vi "ESP32 Continuous Serial Write and Read.vi"() -> ()   [LabVIEW 2021]
doc: "This example performs writes and reads on a serial port, as directed by the user. You can press the Write and Read buttons, and change the Read Count, while the example is running.\n\nThe parameters set for the serial port must match the parameters of the connected instrument or device. In this example, the Read Count parameter specifies the number of bytes that the serial port reads. If there were more bytes at the port than the specified number, those bytes would not be read. If there were less bytes at the port than the specified number, you would receive a timeout error.\n\nThis example expands upon the flow control options for XON and XOFF, allowing the user to choose those control characters. Also, the user can enable or disable a termination character. Some devices require a termination character in order to identify the end of command strings. Some devices send a termination character to signify the end of data to be read. This example shows how you can end the Read operation once a termination character is detected in the buffer and/or append a termination character at the end of the Write data."
uses:
  Program Files (x86)/National Instruments/LabVIEW 2021/examples/Instrument IO/Serial/support/Serial - Settings.ctl
  Program Files (x86)/National Instruments/LabVIEW 2021/examples/Instrument IO/Serial/support/Serial - XON-XOFF Characters.ctl
  Program Files (x86)/National Instruments/LabVIEW 2021/examples/Instrument IO/Serial/support/Serial - ASCII Characters.ctl
  ESP32-PSOC-State Machine.ctl
  <vilib>/Instr/_visa.llb/VISA Flush IO Buffer Mask.ctl
  <vilib>/Instr/_visa.llb/VISA Configure Serial Port (Instr).vi
panel:
  out "error":bool
  out "Connected":bool
  out "Serial Settings:Number of Bytes at Serial Port":u32
  out "Response 2":string
  in  "Command B":bool
  in  "Command A":bool
  in  "Toggle LED":bool
  in  "Enum":T1
  in  "Termination Character":u8=10 format="%.0x"
  in  "End Write on Termination Character?":bool=TRUE
  in  "Stop":bool
  out "Read Count":u32=1000
  out "Response":string
  in  "XON/XOFF Characters":T2={"XON"=enum."DC1", "XOFF"=enum."DC3"}
  in  "Serial Settings":T4={"baud rate"=115200, "data bits"=8, "parity"=enum."None", "stop bits"=10, "flow control"=0} {"flow control" items=["None"=0, "XON/XOFF"=1, "RTS/CTS"=2, "DTR/DSR"=4]; "stop bits" items=["1.0"=10, "1.5"=15, "2.0"=20]; "data bits" min=5 max=8 step=1; "baud rate" items=["75"=75, "110"=110, "134"=134, "150"=150, "300"=300, "600"=600, "1200"=1200, "1800"=1800, "2400"=2400, "4800"=4800, "7200"=7200, "9600"=9600, "14400"=14400, "19200"=19200, "28800"=28800, "38400"=38400, "56000"=56000, "57600"=57600, "115200"=115200, "128000"=128000, "230400"=230400]}
  in  "End Read on Termination Character?":bool=TRUE
  in  "VISA resource name":refnum<visa-resource-name>="COM4"
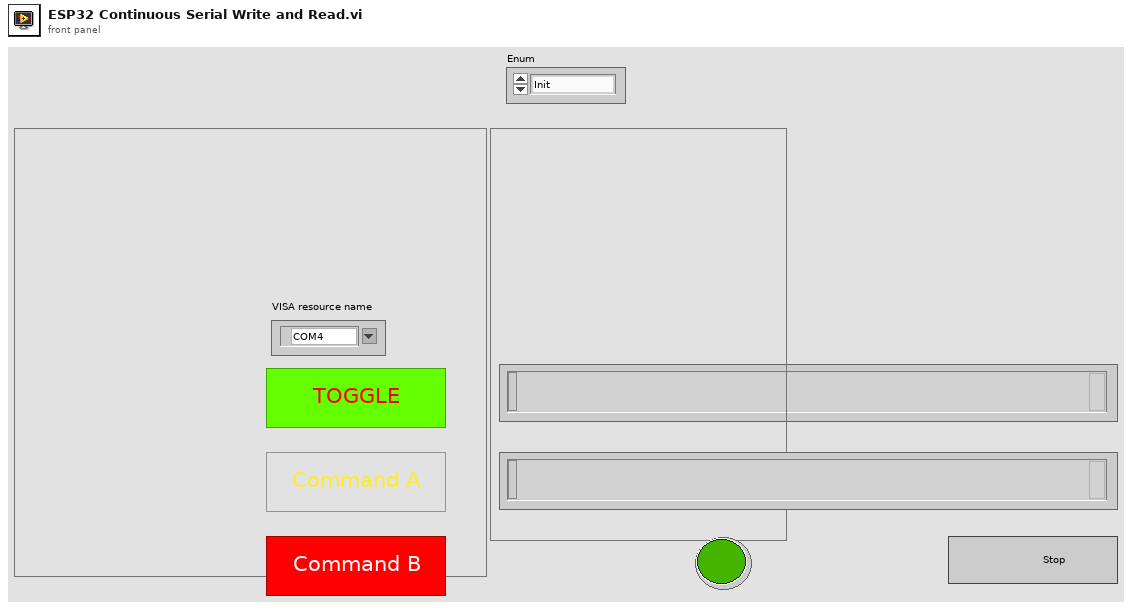
[diagram p1: front panel]
types:
  T1 = typedef "ESP32-PSOC-State Machine.ctl" = enum8{"Init", "Connect", "idle", "send", "wait", "receive", "que", "error", "exit"}
  T2 = typedef "Serial - XON-XOFF Characters.ctl" = cluster{"XON":T3, "XOFF":T3}
  T3 = typedef "Serial - ASCII Characters.ctl" = enum16{"NUL", "SOH", "STX", "ETX", "EOT", "ENQ", "ACK", "BEL", "BS", "HT", "LF", "VT", "FF", "CR", "SO", "SI", "DLE", "DC1", "DC2", "DC3", "DC4", "NAK", "SYN", "ETB", "CAN", "EM", "SUB", "ESC", "FS", "GS", "RS", "US", "SP", "!", "\"", "#", "$", "%", "&", "'", "(", ")", "*", "+", ",", "- (-)", ".", "/", "0", "1", "2", "3", "4", "5", "6", "7", "8", "9", ":", ";", "<", "=", ">", "?", "@", "A", "B", "C", "D", "E", "F", "G", "H", "I", "J", "K", "L", "M", "N", "O", "P", "Q", "R", "S", "T", "U", "V", "W", "X", "Y", "Z", "[", "\\", "]", "^", "_", "`", "a", "b", "c", "d", "e", "f", "g", "h", "i", "j", "k", "l", "m", "n", "o", "p", "q", "r", "s", "t", "u", "v", "w", "x", "y", "z", "{", "|", "}", "~"}
  T4 = typedef "Serial - Settings.ctl" = cluster{"baud rate":u32, "data bits":u16, "parity":enum16{"None", "Odd", "Even", "Mark", "Space"}, "stop bits":u16, "flow control":u16}
  T5 = typedef "VISA Flush IO Buffer Mask.ctl" = u16
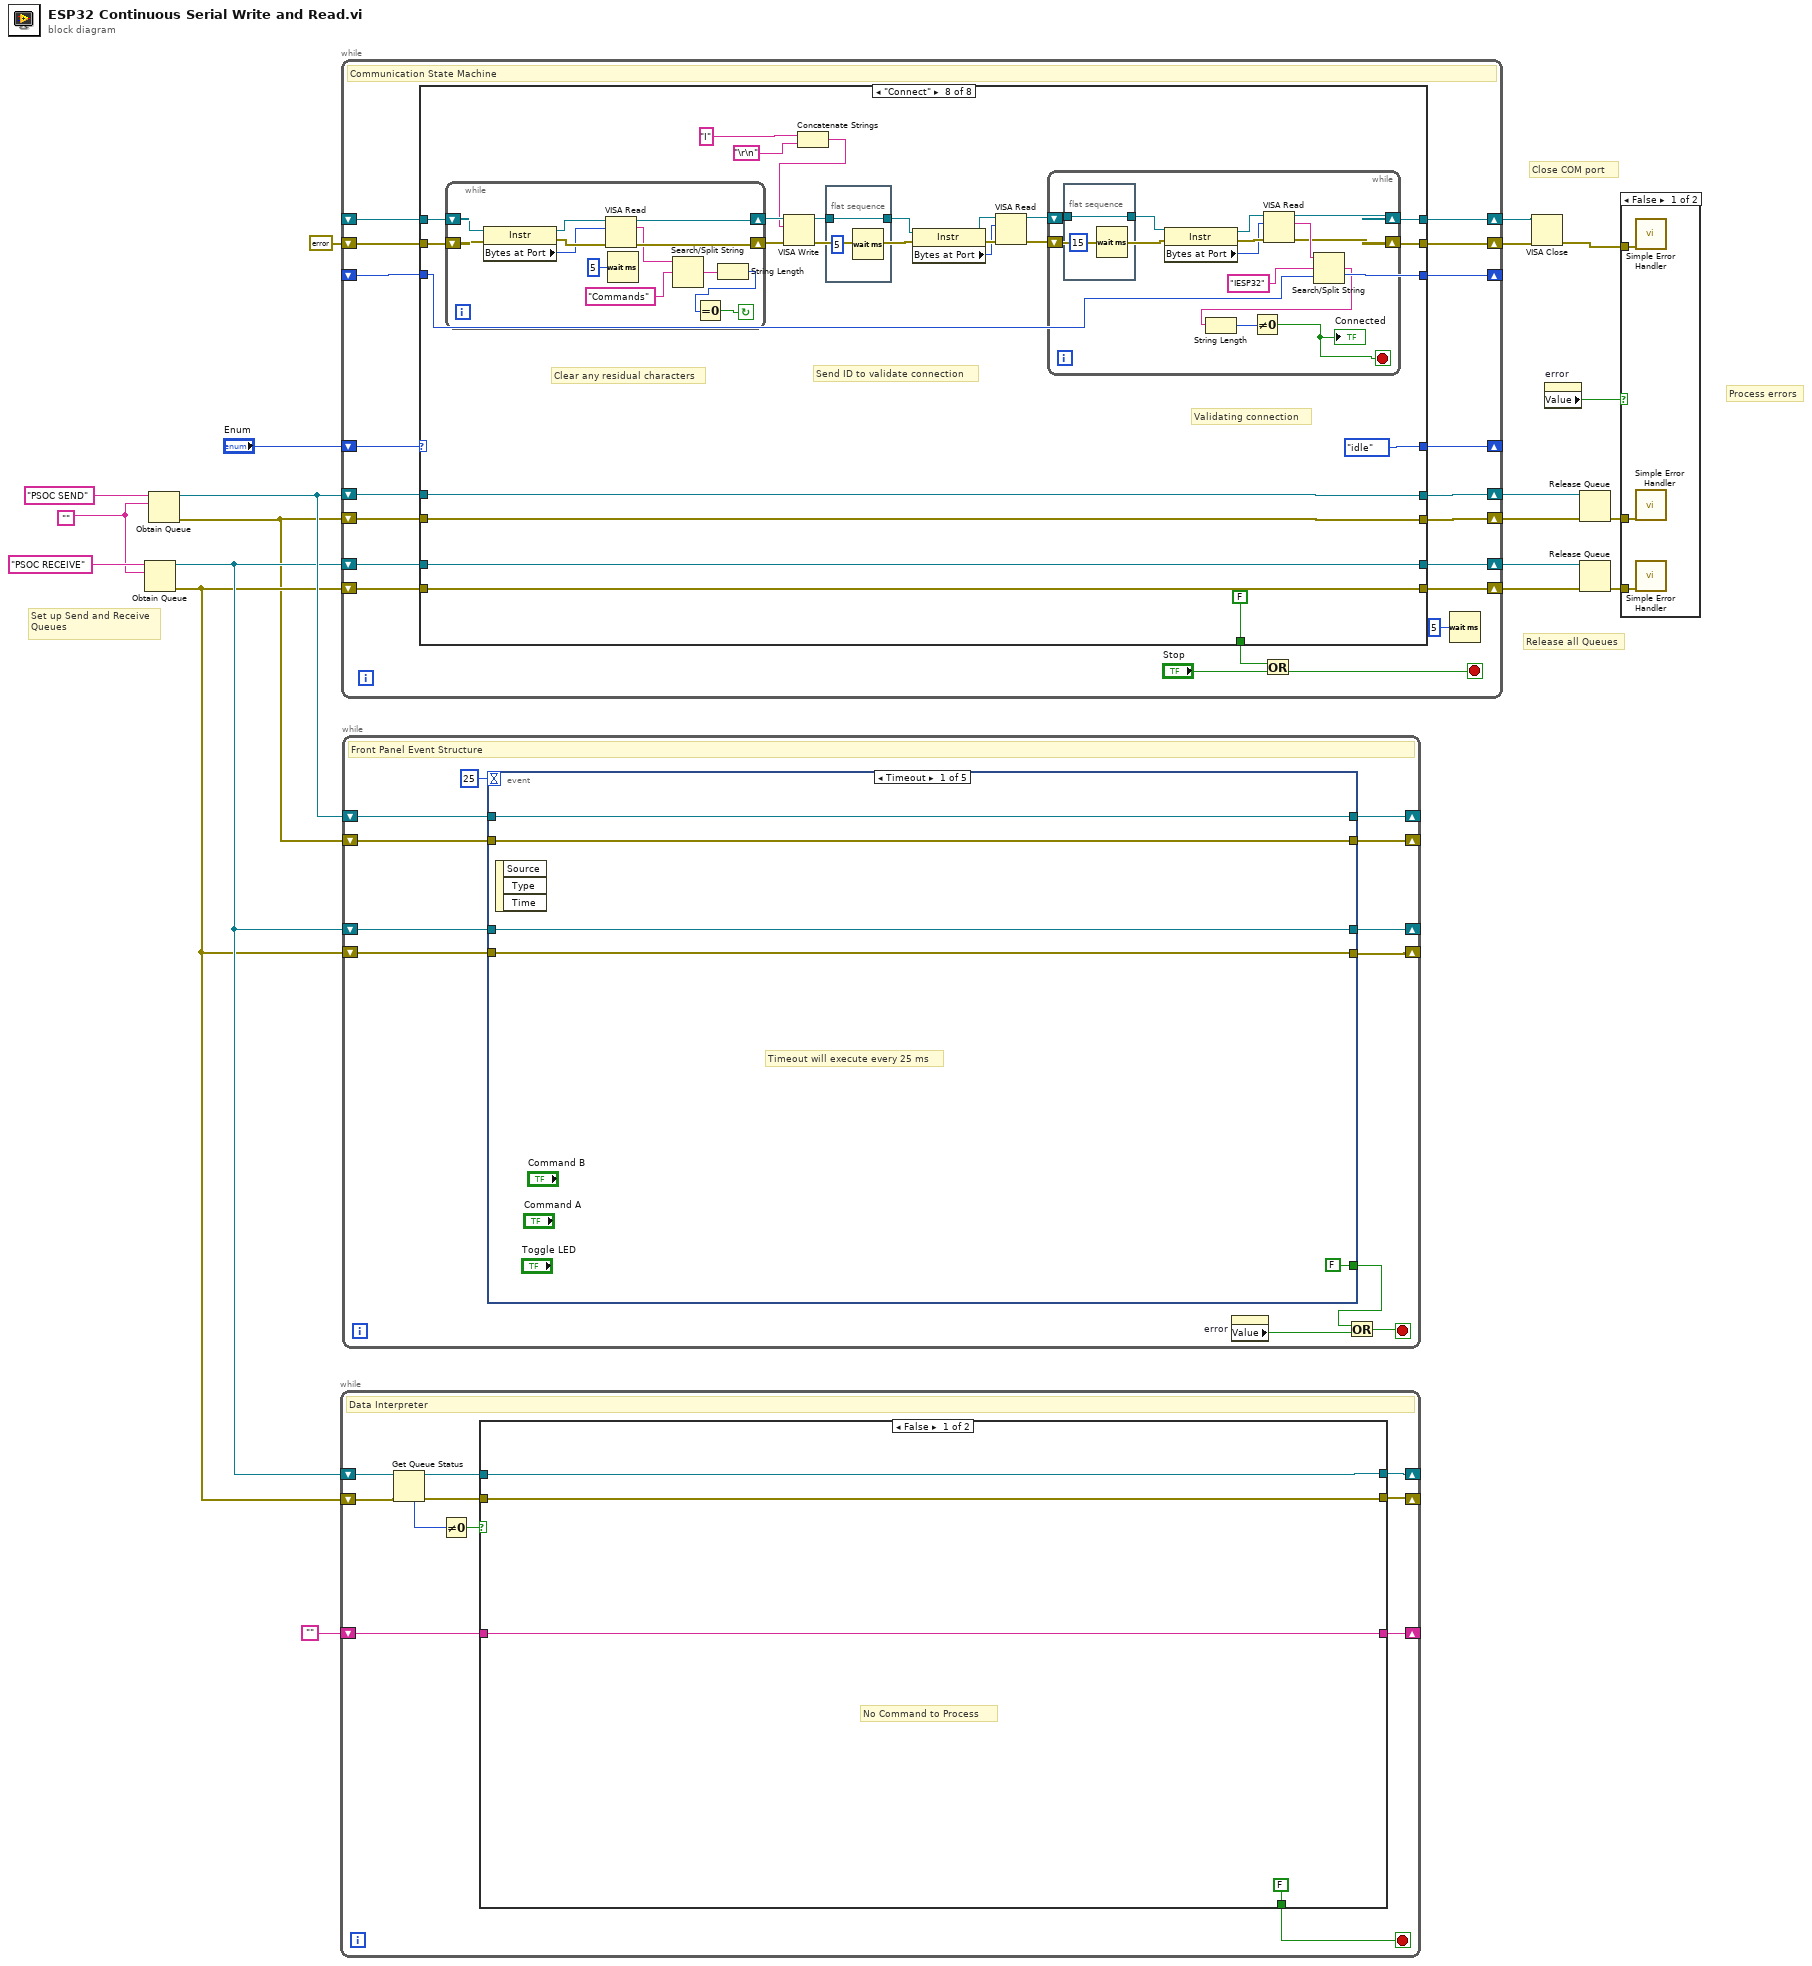
[diagram p0: block diagram]
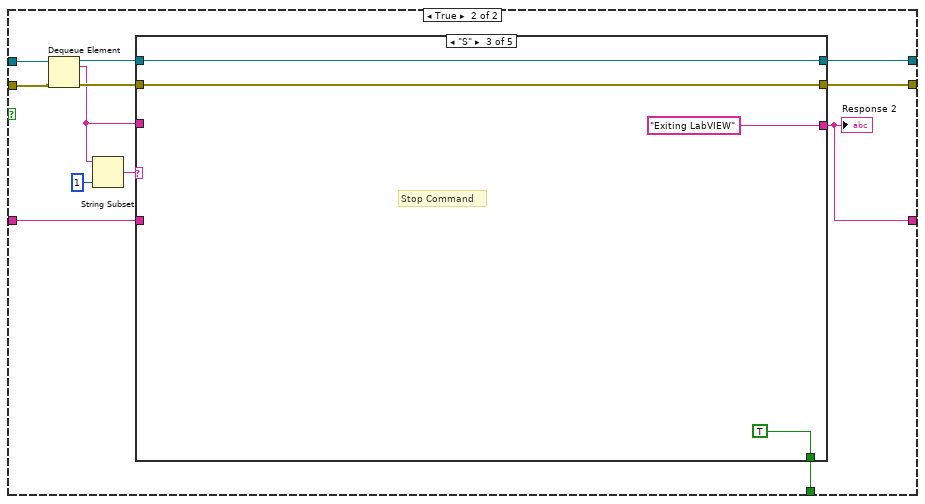
[diagram p3: hidden frame]
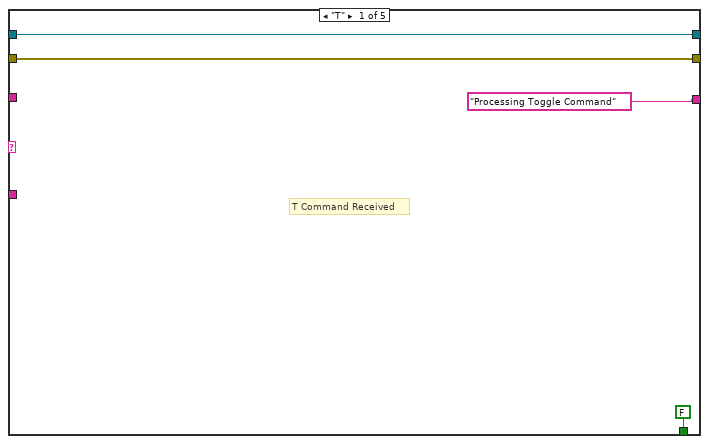
[diagram p4: hidden frame]
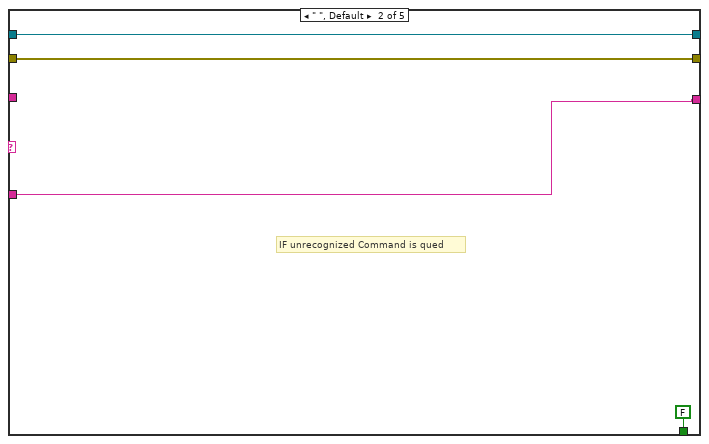
[diagram p5: hidden frame]
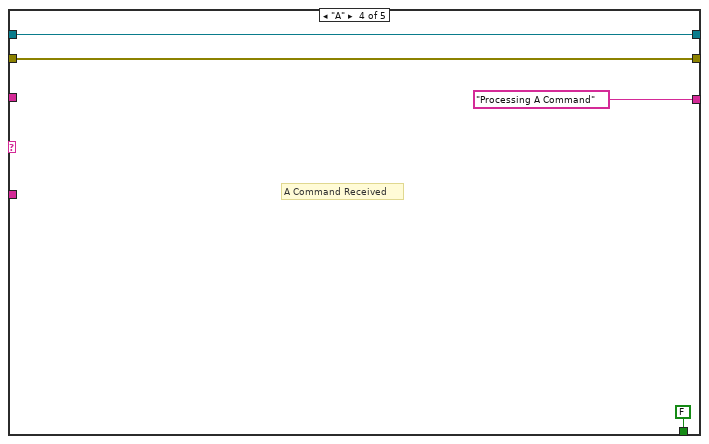
[diagram p6: hidden frame]
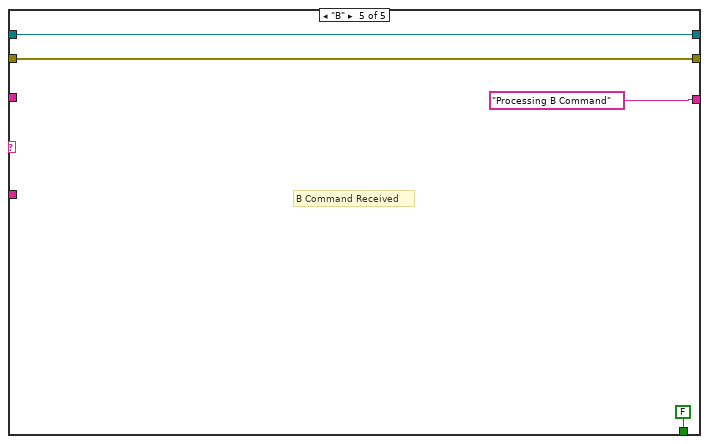
[diagram p7: hidden frame]
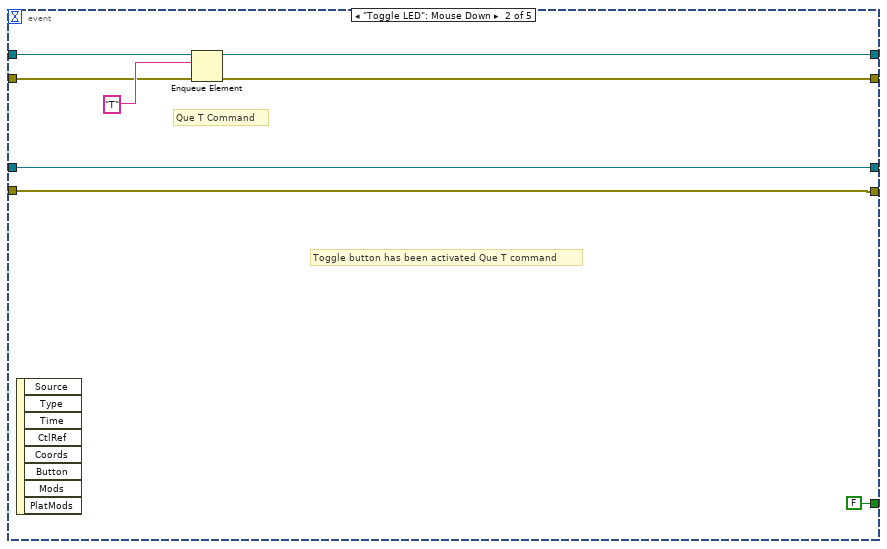
[diagram p8: hidden frame]
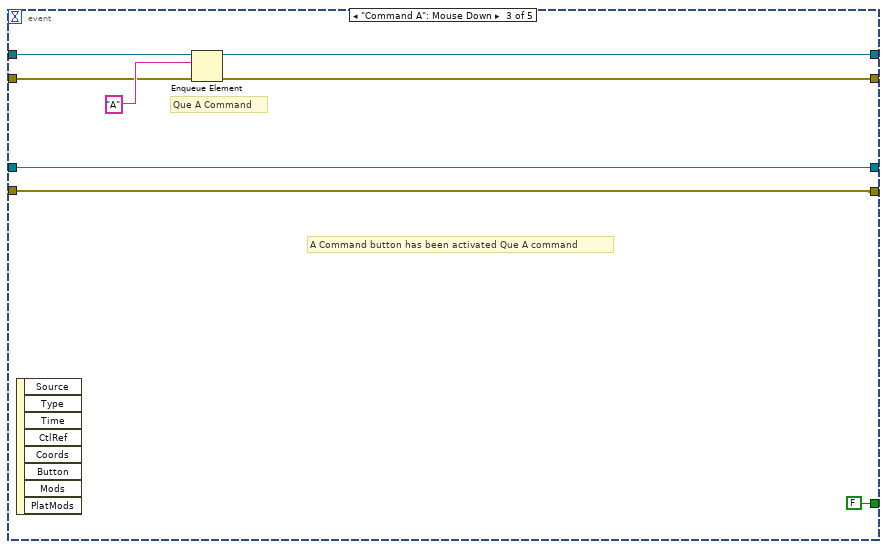
[diagram p9: hidden frame]
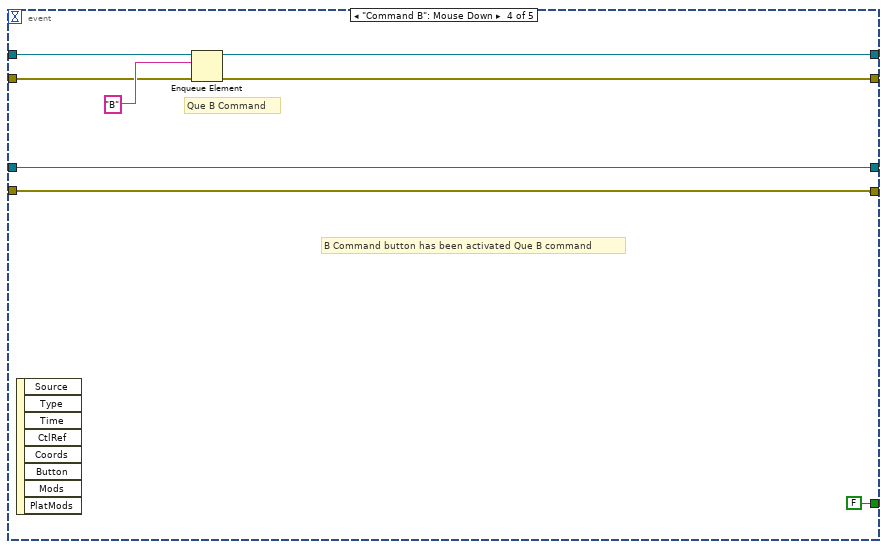
[diagram p10: hidden frame]
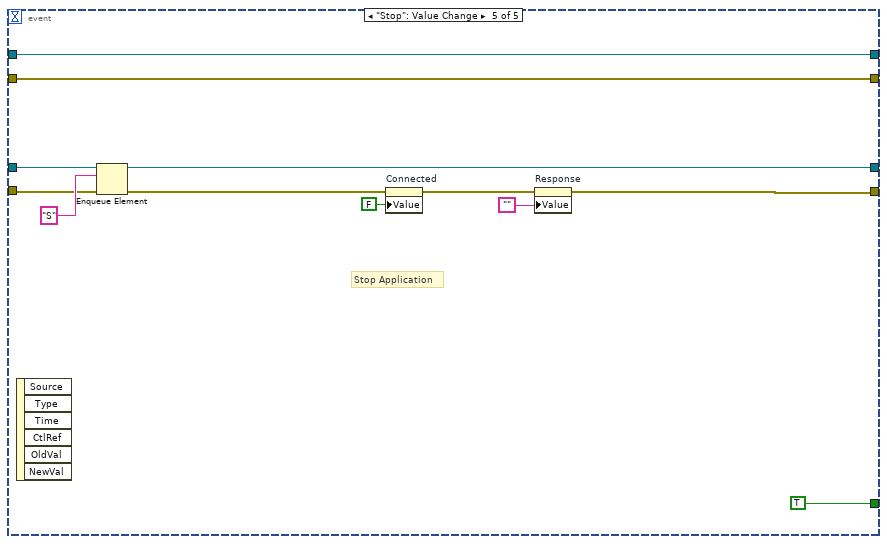
[diagram p11: hidden frame]
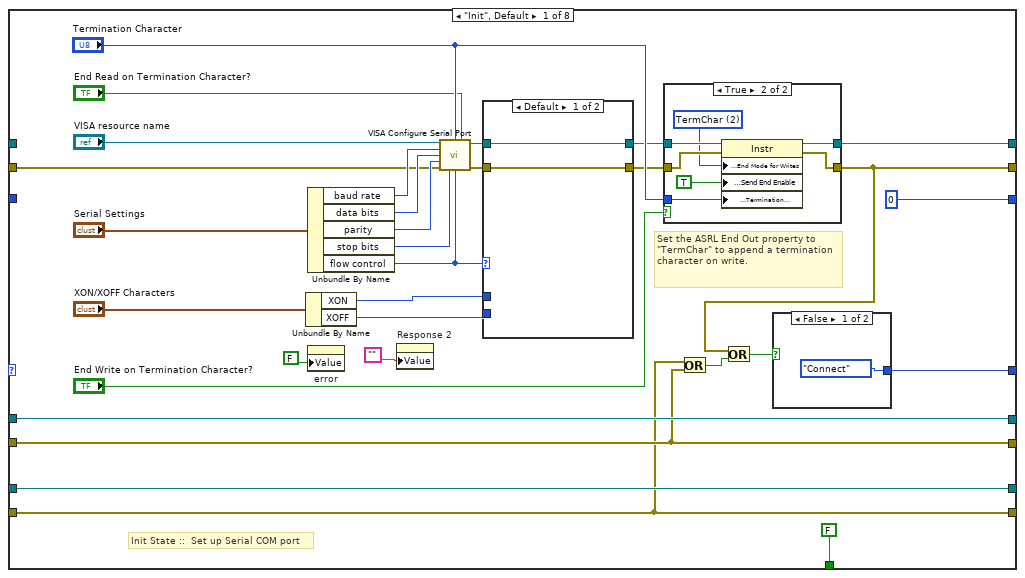
[diagram p12: hidden frame]
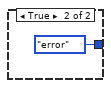
[diagram p13: hidden frame]
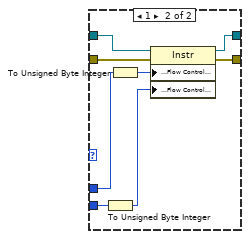
[diagram p15: hidden frame]
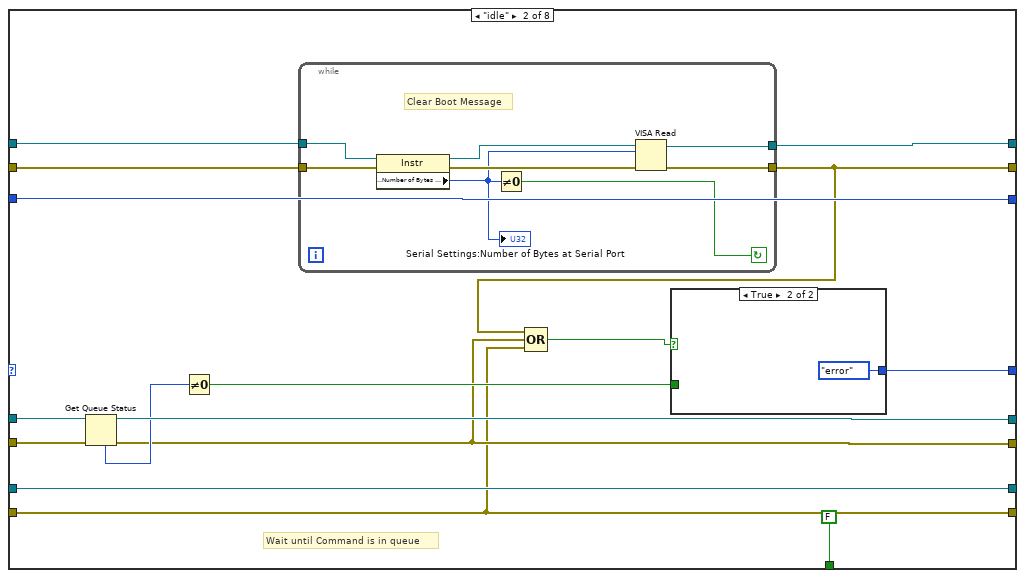
[diagram p16: hidden frame]
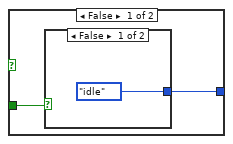
[diagram p17: hidden frame]
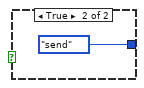
[diagram p18: hidden frame]
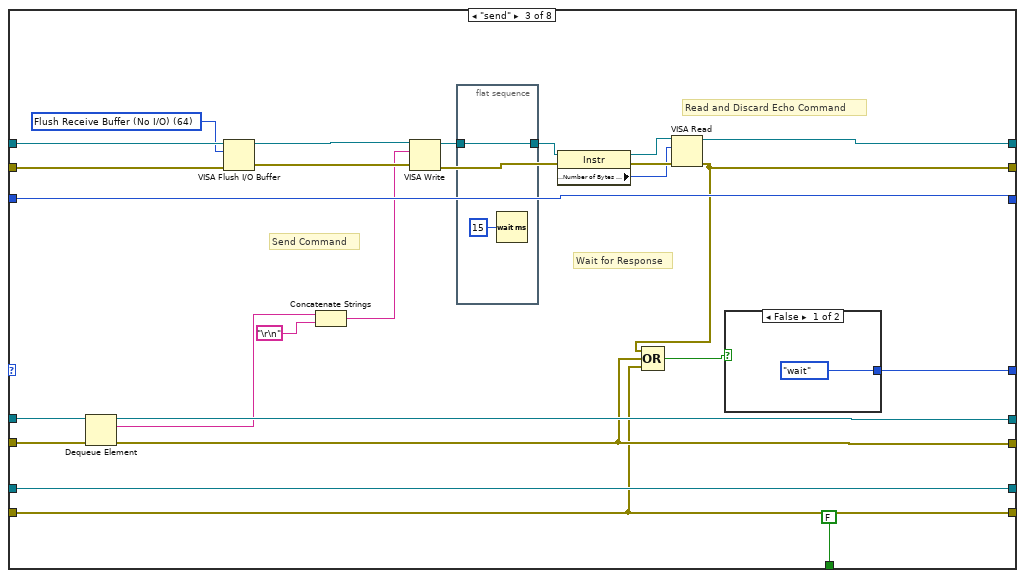
[diagram p19: hidden frame]
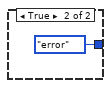
[diagram p20: hidden frame]
diagram:
  w10 = ""
  # "Process errors"
  # "Release all Queues"
  # "Close COM port"
  # "Set up Send and Receive\nQueues"
  n1 = Obtain Queue(name (unnamed)="PSOC RECEIVE", element data type=w10) -> (queue out=w9:refnum<queue>, error out=w8:errorcluster)  [unwired: 3 in, 1 out]
  n2 = Obtain Queue(name (unnamed)="PSOC SEND", element data type=w10) -> (queue out=w12:refnum<queue>, error out=w2:errorcluster)  [unwired: 3 in, 1 out]
  n3 = while {
    shift-right: [w25] -> _
    shift-left: w9 -> [w31]
    shift-right: [w24] -> _
    shift-left: w8 -> [w30]
    shift-right: [w22] -> _
    shift-left: "" -> [w21]
    stop <- w23 stop-if-true
    # "Data Interpreter"
    n4 = Get Queue Status(queue=w31, error in (no error)=w30) -> (queue out=w27:refnum<queue>, error out=w26:errorcluster, # elements in queue=w29:i32)  [unwired: 1 in, 5 out]
    n5 = Not Equal To 0?(x=w29) -> (x != 0?=w28:bool)
    n6 = case shown="False" w28 {
      tunnel: w27 -> [w35 w47]
      tunnel: w26 -> [w34 w46]
      tunnel: [w35 w41] -> w25
      tunnel: [w34 w40] -> w24
      tunnel: [FALSE w39] -> w23
      tunnel: [w32 w37] -> w22
      tunnel: w21 -> [w32 w36]
      frame False {
        # "No Command to Process"
      }
      frame True {
        n7 = Dequeue Element(queue=w47, error in (no error)=w46) -> (queue out=w45:refnum<queue>, element=w38:string, error out=w44:errorcluster)  [unwired: 1 in, 1 out]
        n8 = String Subset(string=w38, length (rest)=1 ("length (rest)")) -> (substring=w42:string)  [unwired: 1 in]
        n9 = case shown="\"S\"" w42 {
          tunnel: w45 -> [w51 w55 w59 w63 w67]
          tunnel: w44 -> [w50 w54 w58 w62 w66]
          tunnel: [w51 w55 w59 w63 w67] -> w41
          tunnel: [w50 w54 w58 w62 w66] -> w40
          tunnel: w38 -> [_ _ _ _ _]
          tunnel: [FALSE FALSE TRUE FALSE FALSE] -> w39
          tunnel: ["Processing Toggle Command" w52 "Exiting LabVIEW" "Processing A Command" "Processing B Command"] -> w37
          tunnel: w36 -> [_ w52 _ _ _]
          frame "T" {
            # "T Command Received"
          }
          frame " ", Default {
            # "IF unrecognized Command is qued"
          }
          frame "S" {
            # "Stop Command"
          }
          frame "A" {
            # "A Command Received"
          }
          frame "B" {
            # "B Command Received"
          }
        }
        "Response 2" <- w37
      }
    }
  }
  n10 = while {
    shift-right: [w79] -> w20
    shift-left: w12 -> [w87]
    shift-right: [w78] -> w18
    shift-left: w2 -> [w86]
    shift-right: [w77] -> w19
    shift-left: w9 -> [w85]
    shift-right: [w76] -> w15
    shift-left: w8 -> [w84]
    shift-right: [w71] -> _
    shift-left: "Enum" -> [w70]
    shift-right: [w83] -> w14
    shift-left: _ -> [w80]
    shift-right: [w82] -> w13
    shift-left: errorcluster {"status"=FALSE, "code"=0, "source"=""} ("error out") -> [w81]
    shift-right: [w75] -> _
    shift-left: _ -> [w74]
    stop <- w69 stop-if-true
    # "Communication State Machine"
    n11 = case shown="\"Connect\"" w70 {
      selector: w70 -> [_ _ _ _ _ _ w287 _]
      tunnel: [w117 w153 w192 w209 w246 w271 w286 w309] -> w79
      tunnel: [w91 w143 w183 w203 w228 w268 w285 w308] -> w78
      tunnel: [w97 w151 w184 w212 w247 ESP32-PSOC-State_Machine."exit" ("Enum") w287 ESP32-PSOC-State_Machine."idle" ("Enum")] -> w71
      tunnel: w87 -> [w117 w155 w194 w209 w246 w271 w286 w309]
      tunnel: w86 -> [w91 w154 w193 w203 w228 w268 w285 w308]
      tunnel: w85 -> [w118 w149 w191 w206 w241 w270 w284 w307]
      tunnel: w84 -> [w90 w142 w182 w202 w227 w267 w275 w306]
      tunnel: [w99 w146 w178 w211 w236 w273 w290 w311] -> w83
      tunnel: [w93 w144 w179 w204 w229 w269 w289 w312] -> w82
      tunnel: w81 -> [w95 w145 w187 w210 w231 w269 w289 w313]
      tunnel: w80 -> [_ w147 w189 w200 w244 w273 w290 w314]
      tunnel: [w118 w149 w191 w206 w239 w270 w282 w307] -> w77
      tunnel: [w90 w142 w182 w202 w240 w267 w278 w306] -> w76
      tunnel: [u32 0 ("Bytes at Port") w148 w190 w208 w242 w272 w288 w310] -> w75
      tunnel: w74 -> [_ w148 w190 _ w238 w272 w288 w310]
      tunnel: [FALSE FALSE FALSE FALSE FALSE FALSE TRUE FALSE] -> w68
      frame "Init", Default {
        # "Init State ::  Set up Serial COM port"
        # "Set the ASRL End Out property to \"TermChar\" to append a termination character on write."
        n12 = Unbundle By Name("XON/XOFF Characters") -> ("XON"=w111:T3, "XOFF"=w112:T3)
        n13 = Unbundle By Name("Serial Settings") -> ("baud rate"=w107:u32, "data bits"=w106:u16, "parity"=w105:enum16{"None", "Odd", "Even", "Mark", "Space"}, "stop bits"=w104:u16, "flow control"=w110:u16)
        n14 = property on="error" class="Bool (strict)"("Value"=FALSE ("error")) -> ()  [unwired: 2 in, 2 out]
        n15 = property on="Response 2" class="Str"("Value"="") -> ()  [unwired: 2 in, 2 out]
        n16 = call-poly "VISA Configure Serial Port"("VISA resource name"="VISA resource name", "termination char\n(0xA = '\\n' = LF)"="Termination Character", "Enable Termination\nChar (T)"="End Read on Termination Character?", "baud rate (9600)"=w107, "data bits (8)"=w106, "parity (0:none)"=w105, "error in (no error)"=w95, "stop bits (10: 1 bit)"=w104, "flow control (0:none)"=w110) -> ("VISA resource name out"=w103:refnum<visa-resource-name>, "error out"=w102:errorcluster)  [unwired: 1 in, 4 out]
        n17 = case shown="Default" w110 {
          tunnel: [w130 w139] -> w113
          tunnel: [w131 w138] -> w114
          tunnel: w102 -> [w130 w137]
          tunnel: w103 -> [w131 w136]
          tunnel: w111 -> [_ w135]
          tunnel: w112 -> [_ w134]
          frame Default {
          }
          frame 1 {
            n18 = To Unsigned Byte Integer(number=w134) -> (unsigned 8bit integer=w133:u8)
            n19 = To Unsigned Byte Integer(number=w135) -> (unsigned 8bit integer=w132:u8)
            n20 = property class="Instr"(reference=w136, error in=w137, "Serial Settings:Flow Control XON Character"=w132, "Serial Settings:Flow Control XOFF Character"=w133) -> (reference out=w138:refnum<visa-resource-name>, error out=w139:errorcluster)
          }
        }
        n21 = case shown="True" "End Write on Termination Character?" {
          tunnel: w114 -> [w121 w129]
          tunnel: w113 -> [w122 w128]
          tunnel: [w121 w127] -> w99
          tunnel: [w122 w126] -> w93
          tunnel: "Termination Character" -> [_ w124]
          frame False {
          }
          frame True {
            w125 = u16 2 items=["None", "LastBit", "TermChar", "Break"] ("Serial Settings:Serial End Mode for Writes")
            n22 = property class="Instr"(reference=w129, error in=w128, "Serial Settings:End Mode for Writes"=w125, "Message Based Settings:Send End Enable"=TRUE, "Message Based Settings:Termination Character"=w124) -> (reference out=w127:refnum<visa-resource-name>, error out=w126:errorcluster)
          }
        }
        n23 = Or(x=w90, y=w91) -> (x .or. y?=w92:bool)
        n24 = Or(x=w93, y=w92) -> (x .or. y?=w94:bool)
        n25 = case shown="False" w94 {
          tunnel: [ESP32-PSOC-State_Machine."Connect" ("Enum") ESP32-PSOC-State_Machine."error" ("Enum")] -> w97
          frame False {
          }
          frame True {
          }
        }
      }
      frame "idle" {
        # "Wait until Command is in queue"
        n26 = Get Queue Status(queue=w155, error in (no error)=w154) -> (queue out=w153:refnum<queue>, error out=w143:errorcluster, # elements in queue=w152:i32)  [unwired: 1 in, 5 out]
        n27 = Not Equal To 0?(x=w152) -> (x != 0?=w150:bool)
        n28 = while {
          tunnel: w147 -> [w168]
          tunnel: [w164] -> w146
          tunnel: w145 -> [w167]
          tunnel: [w162] -> w144
          stop <- w166 continue-if-true
          # "Clear Boot Message"
          n29 = property class="Instr"(reference=w168, error in=w167) -> (reference out=w165:refnum<visa-resource-name>, error out=w163:errorcluster, "Serial Settings:Number of Bytes at Serial Port"=w161:u32)
          "Serial Settings:Number of Bytes at Serial Port" <- w161
          n30 = Not Equal To 0?(x=w161) -> (x != 0?=w166:bool)
          n31 = VISA Read(VISA resource name=w165, byte count=w161, error in (no error)=w163) -> (VISA resource name out=w164:refnum<visa-resource-name>, error out=w162:errorcluster)  [unwired: 2 out]
        }
        n32 = Compound Arithmetic op=OR(w144, w143, w142) -> (w141:bool)
        n33 = case shown="True" w141 {
          tunnel: [w157 ESP32-PSOC-State_Machine."error" ("Enum")] -> w151
          tunnel: w150 -> [w156 _]
          frame False {
            n34 = case shown="False" w156 {
              tunnel: [ESP32-PSOC-State_Machine."idle" ("Enum") ESP32-PSOC-State_Machine."send" ("Enum")] -> w157
              frame False {
              }
              frame True {
              }
            }
          }
          frame True {
          }
        }
      }
      frame "send" {
        w185 = T5 64 items=["Flush Receive Buffer"=16, "Write Transmit Buffer to Device"=32, "Flush Receive Buffer (No I/O)"=64, "Flush Transmit Buffer"=128] ("Mask")
        # "Read and Discard Echo Command"
        # "Wait for Response"
        # "Send Command"
        n35 = Dequeue Element(queue=w194, error in (no error)=w193) -> (queue out=w192:refnum<queue>, element=w172:string, error out=w183:errorcluster)  [unwired: 1 in, 1 out]
        n36 = VISA Flush I/O Buffer(VISA resource name=w189, mask (16)=w185, error in (no error)=w187) -> (VISA resource name out=w188:refnum<visa-resource-name>, error out=w186:errorcluster)
        n37 = Concatenate Strings(w172, "\r\n") -> (w171:string)
        n38 = VISA Write(VISA resource name=w188, write buffer=w171, error in (no error)=w186) -> (VISA resource name out=w170:refnum<visa-resource-name>, error out=w176:errorcluster)  [unwired: 1 out]
        n39 = flat-sequence {
          tunnel: w170 -> [w196]
          tunnel: [w196] -> w169
          frame #0 {
            n40 = Wait (ms)(milliseconds to wait=u32 15) -> ()  [unwired: 1 out]
          }
        }
        n41 = property class="Instr"(reference=w169, error in=w176) -> (reference out=w177:refnum<visa-resource-name>, error out=w175:errorcluster, "Serial Settings:Number of Bytes at Serial Port"=w174:u32)
        n42 = VISA Read(VISA resource name=w177, byte count=w174, error in (no error)=w175) -> (VISA resource name out=w178:refnum<visa-resource-name>, error out=w179:errorcluster)  [unwired: 2 out]
        n43 = Compound Arithmetic op=OR(w179, w183, w182) -> (w181:bool)
        n44 = case shown="False" w181 {
          tunnel: [ESP32-PSOC-State_Machine."wait" ("Enum") ESP32-PSOC-State_Machine."error" ("Enum")] -> w184
          frame False {
          }
          frame True {
          }
        }
      }
      frame "wait" {
        # "Wait for actual Response"
        n45 = flat-sequence {
          tunnel: w200 -> [w214]
          tunnel: [w214] -> w199
          frame #0 {
            n46 = Wait (ms)(milliseconds to wait=u32 15) -> ()  [unwired: 1 out]
          }
        }
        n47 = property class="Instr"(reference=w199, error in=w210) -> (reference out=w211:refnum<visa-resource-name>, error out=w204:errorcluster, "Serial Settings:Number of Bytes at Serial Port"=w208:u32)
        n48 = Not Equal To 0?(x=w208) -> (x != 0?=w207:bool)
        n49 = Compound Arithmetic op=OR(w204, w203, w202) -> (w205:bool)
        n50 = case shown="False" w205 {
          tunnel: [w216 ESP32-PSOC-State_Machine."error" ("Enum")] -> w212
          tunnel: w207 -> [w215 _]
          frame False {
            n51 = case shown="True" w215 {
              tunnel: [ESP32-PSOC-State_Machine."wait" ("Enum") ESP32-PSOC-State_Machine."receive" ("Enum")] -> w216
              frame False {
              }
              frame True {
              }
            }
          }
          frame True {
          }
        }
      }
      frame "receive" {
        # "Process Response and Display"
        # "Read Response"
        n52 = VISA Read(VISA resource name=w244, byte count=w238, error in (no error)=w231) -> (VISA resource name out=w237:refnum<visa-resource-name>, read buffer=w233:string, error out=w243:errorcluster)  [unwired: 1 out]
        n53 = String To Byte Array(string=w233) -> (unsigned byte array=w232:u8[])
        n54 = property class="Instr"(reference=w237, error in=w243) -> (reference out=w236:refnum<visa-resource-name>, error out=w230:errorcluster, "Serial Settings:Number of Bytes at Serial Port"=w242:u32)
        n55 = Index Array(array=w232, index=0) -> (element=w224:u8)
        n56 = Equal?(x=w224, y=u8 13) -> (x = y?=w222:bool)
        n57 = Equal?(x=w224, y=u8 10) -> (x = y?=w221:bool)
        n58 = Not Or(1:w221, 2:w222) -> (0:w220:bool)
        n59 = Not Equal To 0?(x=w242) -> (x != 0?=w245:bool)
        n60 = case shown="True" w220 {
          tunnel: w232 -> [_ w262]
          tunnel: w230 -> [w253 w255]
          tunnel: [w253 w254] -> w229
          frame False {
          }
          frame True {
            n61 = Delete From Array(array=w262, length=1, index=0) -> (array with subset deleted=w259:u8[])  [unwired: 1 out]
            n62 = property on="Response" class="Str"(error in=w255, "Value"="") -> (error out=w257:errorcluster)  [unwired: 1 in, 1 out]
            n63 = Byte Array To String(unsigned byte array=w259) -> (string=w256:string)
            n64 = property on="Response" class="Str"(error in=w257, "Value"=w256) -> (error out=w254:errorcluster)  [unwired: 1 in, 1 out]
          }
        }
        n65 = Compound Arithmetic op=OR(w229, w228, w227) -> (w226:bool)
        n66 = Enqueue Element(queue=w241, element=w233, error in (no error)=w227) -> (queue out=w239:refnum<queue>, error out=w240:errorcluster)  [unwired: 1 in, 1 out]
        n67 = case shown="False" w226 {
          tunnel: [w249 ESP32-PSOC-State_Machine."error" ("Enum")] -> w247
          tunnel: w245 -> [w248 _]
          frame False {
            n68 = case shown="False" w248 {
              tunnel: [ESP32-PSOC-State_Machine."idle" ("Enum") ESP32-PSOC-State_Machine."receive" ("Enum")] -> w249
              frame False {
              }
              frame True {
              }
            }
          }
          frame True {
          }
        }
        "Read Count" <- w238
      }
      frame "error" {
        # "Process any error"
        n69 = Build Array(w269, w268, w267) -> (w266:errorcluster[])
        n70 = for {
          tunnel: w266 -> [w274] mode=indexing
          n71 = call <vilib>:"General Error Handler.vi"("error in (no error)"=w274) -> ()  [unwired: 10 in, 5 out]
        }
        "error" <- TRUE ("error")
      }
      frame "exit" {
        # "Exit due to error"
        n72 = Enqueue Element(queue=w284, element="S", error in (no error)=w275) -> (queue out=w282:refnum<queue>, error out=w280:errorcluster)  [unwired: 1 in, 1 out]
        n73 = property on="Connected" class="Bool (strict)"(error in=w280, "Value"=FALSE ("Connected")) -> (error out=w279:errorcluster)  [unwired: 1 in, 1 out]
        n74 = property on="Response" class="Str"(error in=w279, "Value"="") -> (error out=w278:errorcluster)  [unwired: 1 in, 1 out]
      }
      frame "Connect" {
        # "Validating connection"
        # "Send ID to validate connection"
        # "Clear any residual characters"
        n75 = while {
          shift-right: [w338] -> w302
          shift-left: w313 -> [w344]
          shift-right: [w337] -> w303
          shift-left: w314 -> [w343]
          stop <- w342 continue-if-true
          n76 = property class="Instr"(reference=w343, error in=w344) -> (reference out=w340:refnum<visa-resource-name>, error out=w339:errorcluster, "Bytes at Port"=w336:u32)
          n77 = VISA Read(VISA resource name=w340, byte count=w336, error in (no error)=w339) -> (VISA resource name out=w337:refnum<visa-resource-name>, read buffer=w335:string, error out=w338:errorcluster)  [unwired: 1 out]
          n78 = Wait (ms)(milliseconds to wait=u32 5) -> ()  [unwired: 1 out]
          n79 = Search/Split String(string=w335, search string/char (-)="Commands") -> (match + rest of string=w333:string)  [unwired: 1 in, 2 out]
          n80 = String Length(string=w333) -> (length=w332:i32)
          n81 = Equal To 0?(x=w332) -> (x = 0?=w342:bool)
        }
        n82 = Concatenate Strings("I" ("write buffer"), "\r\n") -> (w291:string)
        n83 = VISA Write(VISA resource name=w303, write buffer=w291, error in (no error)=w302) -> (VISA resource name out=w297:refnum<visa-resource-name>, error out=w301:errorcluster)  [unwired: 1 out]
        n84 = flat-sequence {
          tunnel: w297 -> [w331]
          tunnel: [w331] -> w296
          frame #0 {
            n85 = Wait (ms)(milliseconds to wait=u32 5) -> ()  [unwired: 1 out]
          }
        }
        n86 = property class="Instr"(reference=w296, error in=w301) -> (reference out=w299:refnum<visa-resource-name>, error out=w300:errorcluster, "Bytes at Port"=w298:u32)
        n87 = VISA Read(VISA resource name=w299, byte count=w298, error in (no error)=w300) -> (VISA resource name out=w294:refnum<visa-resource-name>, error out=w295:errorcluster)  [unwired: 2 out]
        n88 = while {
          shift-right: [w318] -> w312
          shift-left: w295 -> [w324]
          shift-right: [w319] -> w311
          shift-left: w294 -> [w317]
          stop <- w315 stop-if-true
          n89 = flat-sequence {
            tunnel: w317 -> [w329]
            tunnel: [w329] -> w316
            frame #0 {
              n90 = Wait (ms)(milliseconds to wait=u32 15) -> ()  [unwired: 1 out]
            }
          }
          n91 = property class="Instr"(reference=w316, error in=w324) -> (reference out=w322:refnum<visa-resource-name>, error out=w323:errorcluster, "Bytes at Port"=w321:u32)
          n92 = VISA Read(VISA resource name=w322, byte count=w321, error in (no error)=w323) -> (VISA resource name out=w319:refnum<visa-resource-name>, read buffer=w320:string, error out=w318:errorcluster)  [unwired: 1 out]
          n93 = Search/Split String(string=w320, search string/char (-)="IESP32") -> (match + rest of string=w326:string)  [unwired: 1 in, 2 out]
          n94 = String Length(string=w326) -> (length=w325:i32)
          n95 = Not Equal To 0?(x=w325) -> (x != 0?=w315:bool)
          "Connected" <- w315
        }
      }
    }
    n96 = Or(x=w68, y="Stop") -> (x .or. y?=w69:bool)
    n97 = Wait (ms)(milliseconds to wait=u32 5) -> ()  [unwired: 1 out]
  }
  n98 = while {
    shift-right: [w353] -> _
    shift-left: w12 -> [w354]
    shift-right: [w352] -> _
    shift-left: w2 -> [w355]
    shift-right: [w348] -> _
    shift-left: w9 -> [w351]
    shift-right: [w349] -> _
    shift-left: w8 -> [w350]
    stop <- w345 stop-if-true
    # "Front Panel Event Structure"
    n99 = event shown="[0] Timeout" {
      selector: _ -> [_ _ _ _ _]
      dyn-events: _ -> [_ _ _ _ _]
      timeout: 25 -> [_ _ _ _ _]
      tunnel: w355 -> [w359 w367 w375 w383 w395]
      tunnel: w354 -> [w360 w369 w377 w385 w396]
      tunnel: [w360 w366 w374 w382 w396] -> w353
      tunnel: [w359 w365 w373 w381 w395] -> w352
      tunnel: [FALSE FALSE FALSE FALSE TRUE] -> w347
      tunnel: w351 -> [w358 w363 w371 w379 w394]
      tunnel: w350 -> [w357 w362 w370 w378 w392]
      tunnel: [w357 w362 w370 w378 w387] -> w349
      tunnel: [w358 w363 w371 w379 w391] -> w348
      event Timeout {
        # "Timeout will execute every 25 ms"
        n100 = event-data() -> ()  [unwired: 1 in, 3 out]
      }
      event "Toggle LED": Mouse Down {
        # "Que T Command"
        # "Toggle button has been activated Que T command"
        n101 = event-data() -> ()  [unwired: 1 in, 8 out]
        n102 = Enqueue Element(queue=w369, element="T", error in (no error)=w367) -> (queue out=w366:refnum<queue>, error out=w365:errorcluster)  [unwired: 1 in, 1 out]
      }
      event "Command A": Mouse Down {
        # "Que A Command"
        # "A Command button has been activated Que A command"
        n103 = event-data() -> ()  [unwired: 1 in, 8 out]
        n104 = Enqueue Element(queue=w377, element="A", error in (no error)=w375) -> (queue out=w374:refnum<queue>, error out=w373:errorcluster)  [unwired: 1 in, 1 out]
      }
      event "Command B": Mouse Down {
        # "Que B Command"
        # "B Command button has been activated Que B command"
        n105 = event-data() -> ()  [unwired: 1 in, 8 out]
        n106 = Enqueue Element(queue=w385, element="B", error in (no error)=w383) -> (queue out=w382:refnum<queue>, error out=w381:errorcluster)  [unwired: 1 in, 1 out]
      }
      event "Stop": Value Change {
        # "Stop Application"
        n107 = event-data() -> ()  [unwired: 1 in, 6 out]
        n108 = Enqueue Element(queue=w394, element="S", error in (no error)=w392) -> (queue out=w391:refnum<queue>, error out=w390:errorcluster)  [unwired: 1 in, 1 out]
        n109 = property on="Connected" class="Bool (strict)"(error in=w390, "Value"=FALSE ("Connected")) -> (error out=w388:errorcluster)  [unwired: 1 in, 1 out]
        n110 = property on="Response" class="Str"(error in=w388, "Value"="") -> (error out=w387:errorcluster)  [unwired: 1 in, 1 out]
      }
    }
    n111 = property on="error" class="Bool (strict)"() -> ("Value"=w346:bool)  [unwired: 2 in, 2 out]
    n112 = Or(x=w347, y=w346) -> (x .or. y?=w345:bool)
  }
  n113 = VISA Close(VISA resource name=w14, error in (no error)=w13) -> (error out=w5:errorcluster)
  n114 = property on="error" class="Bool (strict)"() -> ("Value"=w1:bool)  [unwired: 2 in, 2 out]
  n115 = Release Queue(queue=w20, error in (no error)=w18) -> (error out=w4:errorcluster)  [unwired: 1 in, 2 out]
  n116 = Release Queue(queue=w19, error in (no error)=w15) -> (error out=w3:errorcluster)  [unwired: 1 in, 2 out]
  n117 = case shown="False" w1 {
    tunnel: w5 -> [w400 _]
    tunnel: w4 -> [w399 _]
    tunnel: w3 -> [w398 _]
    frame False {
      n118 = call <vilib>:"Simple Error Handler.vi"("error in (no error)"=w400) -> ()  [unwired: 1 in, 8 out]
      n119 = call <vilib>:"Simple Error Handler.vi"("error in (no error)"=w399) -> ()  [unwired: 1 in, 8 out]
      n120 = call <vilib>:"Simple Error Handler.vi"("error in (no error)"=w398) -> ()  [unwired: 1 in, 8 out]
    }
    frame True {
    }
  }
